vi "Track Subscriber.vi"(8 "error in (no error)":errorcluster, 10 "SubscriptionRequest":refnum<class "SubscriptionRequest.lvclass">, 11 "IBusMonitor In":refnum<class "IBusMonitor.lvclass">) -> (0 "error out":errorcluster, 3 "IBusMonitor Out":refnum<class "IBusMonitor.lvclass">)   [LabVIEW 2017, in "MonitoredMediator.lvlib" / "IBusMonitor.lvclass"]
uses:
  IBusMonitor.lvclass
  IMediator/SubscriptionRequest/SubscriptionRequest.lvclass
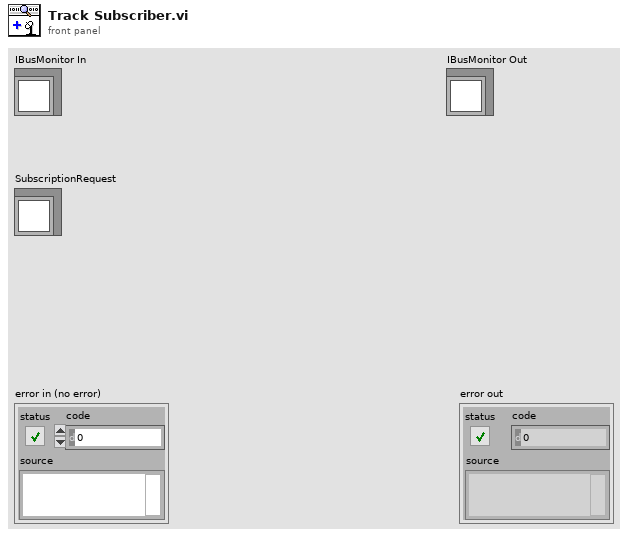
[diagram p1: front panel]
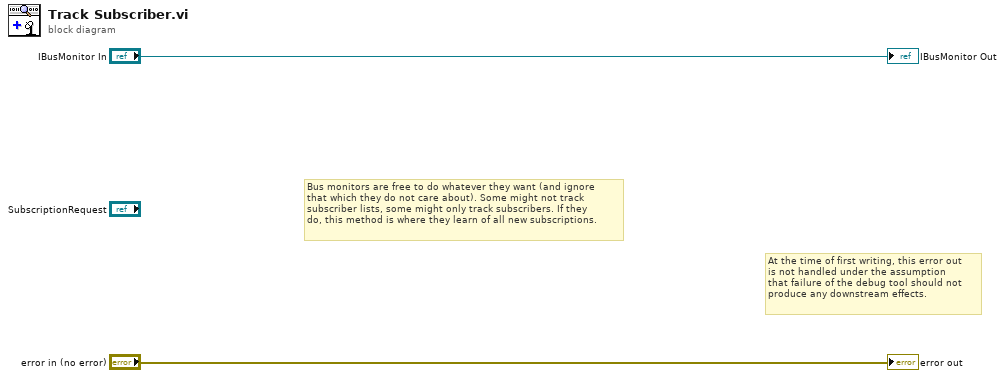
[diagram p0: block diagram]
diagram:
  # "At the time of first writing, this error out\nis not handled under the assumption\nthat failure of the debug tool should not\nproduce any downstream effects."
  # "Bus monitors are free to do whatever they want (and ignore\nthat which they do not care about). Some might not track\nsubscriber lists, some might only track subscribers. If they\ndo, this method is where they learn of all new subscriptions."
  "error out" <- "error in (no error)"
  "IBusMonitor Out" <- "IBusMonitor In"
